vi "moveTo_abs_XYZ_forMJump.vi"(7 "blocking?":bool, 8 "error in":errorcluster, 10 "XYZ location (steps)":i32[](array[numeric]), 11 "Actuator cluster in":T1={"Actuator COM"="COM6", "Actuator type"=enum."Scientifica"}) -> (0 "error out":errorcluster, 3 "Actuator cluster out":T1={"Actuator COM"="COM14", "Actuator type"=enum."Scientifica"})   [LabVIEW 2019]
uses:
  controls/actuator_cluster.ctl
  controls/actuator_type.ctl
  controls/scientifica_commands.ctl
panel:
  out "response":string
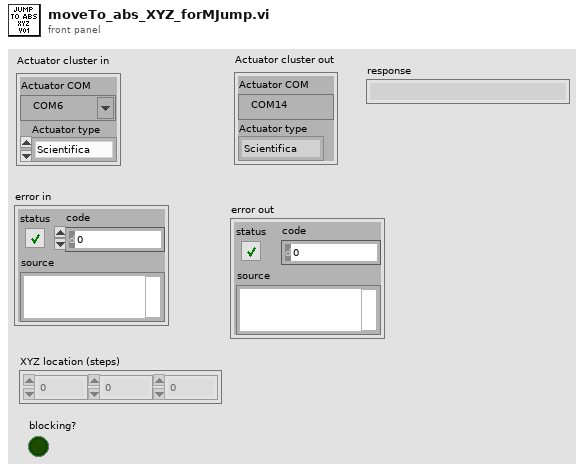
[diagram p1: front panel]
types:
  T1 = typedef "actuator_cluster.ctl" = cluster{"Actuator COM":refnum<visa-resource-name>, "Actuator type":T2}
  T2 = typedef "actuator_type.ctl" = enum16{"Scientifica", "Sutter", "Demo", "Off"}
  T3 = typedef "scientifica_commands.ctl" = enum16{"ANGLE", "INSET", "FIRST", "ZERO", "Pz", "P", "absz", "ACC", "TOP", "STOP", "rel", "relz", "abs", "IN", "vj", "APROACH", "OBJS", "OBJU", "OUT", "OBJ", "OBJL", "SET", "OBJD", "STEP", "SETSTEP", "S", "UUX", "UUY", "UUZ"}
  T4 = enum16{"READY", "ABSOLUTE MOVE", "RELATIVE MOVE", "HOMING", "WAITING", "CANCELING"}
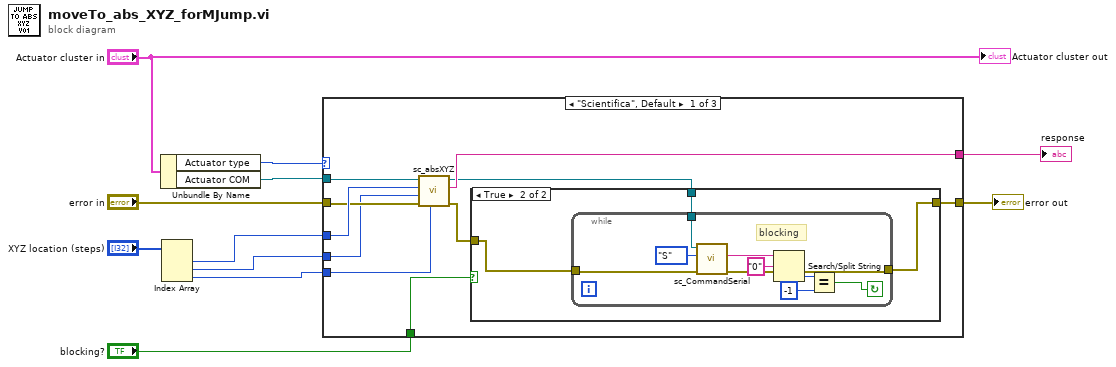
[diagram p0: block diagram]
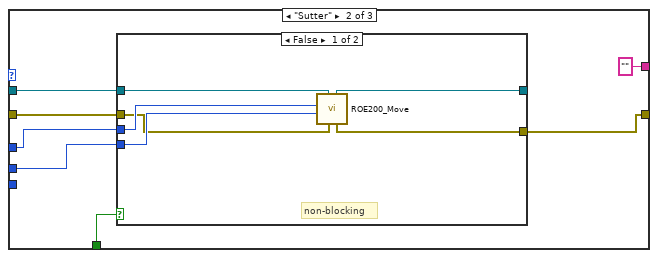
[diagram p3: hidden frame]
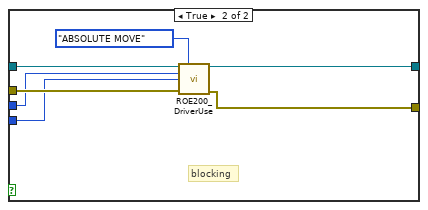
[diagram p4: hidden frame]
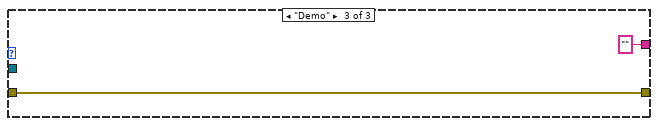
[diagram p5: hidden frame]
diagram:
  n1 = Unbundle By Name("Actuator cluster in") -> ("Actuator type"=w11:T2, "Actuator COM"=w9:refnum<visa-resource-name>)
  n2 = Index Array(array="XYZ location (steps)") -> (element #1=w4:i32, element #2=w3:i32, element #3=w1:i32)  [unwired: 3 in]
  n3 = case shown="\"Scientifica\", Default" w11 {
    tunnel: "error in" -> [w19 w40 w55]
    tunnel: w9 -> [w21 w41 _]
    tunnel: [w14 w36 w55] -> w7
    tunnel: w4 -> [w20 w39 _]
    tunnel: w3 -> [w18 w37 _]
    tunnel: [w17 "" ("argument integer string") "" ("argument integer string")] -> w6
    tunnel: "blocking?" -> [w16 w38 _]
    tunnel: w1 -> [w12 _ _]
    frame "Scientifica", Default {
      n4 = call "sc_absXYZ.vi"("abs Z (steps)"=w12, "error in (no error)"=w19, "abs Y (steps)"=w18, "abs X (steps)"=w20, "VISA handle"=w21) -> ("error out"=w15:errorcluster, "argument integer string"=w17:string, "Dup. VISA handle"=w13:refnum<visa-resource-name>)  [unwired: 4 in]
      n5 = case shown="True" w16 {
        tunnel: w15 -> [w22 w25]
        tunnel: [w22 w24] -> w14
        tunnel: w13 -> [_ w23]
        frame False {
        }
        frame True {
          n6 = while {
            tunnel: w25 -> [w33]
            tunnel: [w27] -> w24
            tunnel: w23 -> [w26]
            stop <- w28 continue-if-true
            # "blocking"
            n7 = call "sc_CommandSerial.vi"("error in (no error)"=w33, "Scientifica commands"=scientifica_commands."S", "VISA handle"=w26) -> ("error out"=w27:errorcluster, "Response"=w31:string)  [unwired: 5 in, 2 out]
            n8 = Search/Split String(string=w31, search string/char (-)="0") -> (offset of match=w30:i32)  [unwired: 1 in, 2 out]
            n9 = Equal?(x=w30, y=-1) -> (x = y?=w28:bool)
          }
        }
      }
    }
    frame "Sutter" {
      n10 = case shown="False" w38 {
        tunnel: w41 -> [w47 w54]
        tunnel: w40 -> [w43 w53]
        tunnel: w39 -> [w46 w52]
        tunnel: w37 -> [w45 w51]
        tunnel: [w44 w49] -> _
        tunnel: [w42 w48] -> w36
        frame False {
          # "non-blocking"
          n11 = call "ROE200_Move.vi"("error in (no error)"=w43, "VISA resource name 2"=w47, "Y"=w45, "X"=w46) -> ("error out"=w42:errorcluster, "VISA resource name out"=w44:refnum<visa-resource-name>)  [unwired: 6 in]
        }
        frame True {
          # "blocking"
          n12 = call "ROE200_DriverUse.vi"("VISA resource name In"=w54, "CMD"=T4."ABSOLUTE MOVE", "X"=w52, "Y"=w51, "error in"=w53) -> ("VISA resource name out"=w49:refnum<visa-resource-name>, "error out"=w48:errorcluster)  [unwired: 6 in, 3 out]
        }
      }
    }
    frame "Demo" {
    }
  }
  "error out" <- w7
  "response" <- w6
  "Actuator cluster out" <- "Actuator cluster in"
